vi "Untitled 1.vi"() -> ()   [LabVIEW 2020]
panel:
  in  "Einzel":dbl(slide) scale=0.0..-10000.0
  in  "wisman test":dbl(slide) scale=0.0..10000.0
  in  "stop":bool
  out "einzel":dbl(graph)
  out "Einzel readback":dbl
  out "wisman":dbl(graph)
  out "readback":dbl
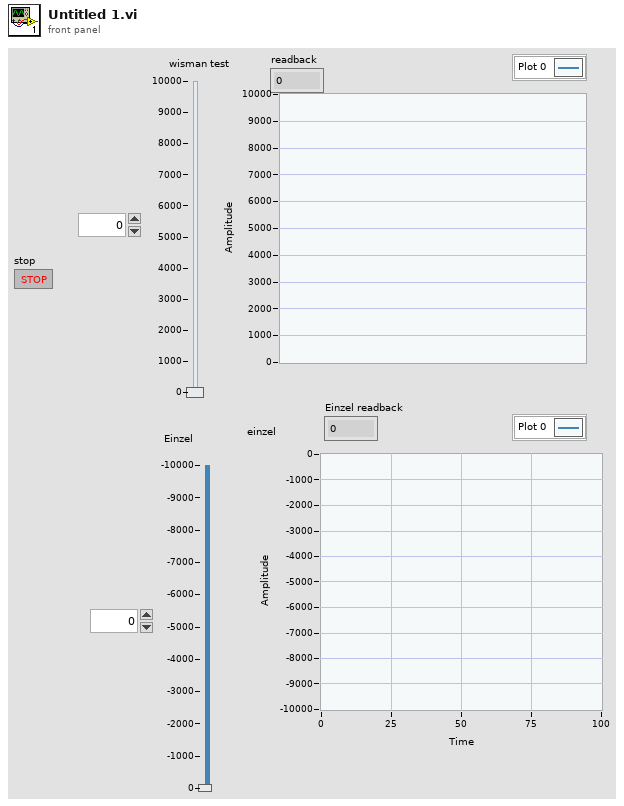
[diagram p1: front panel]
types:
  T1 = enum16{"open", "replace", "create", "open or create", "replace or create", "replace or create with confirmation"}
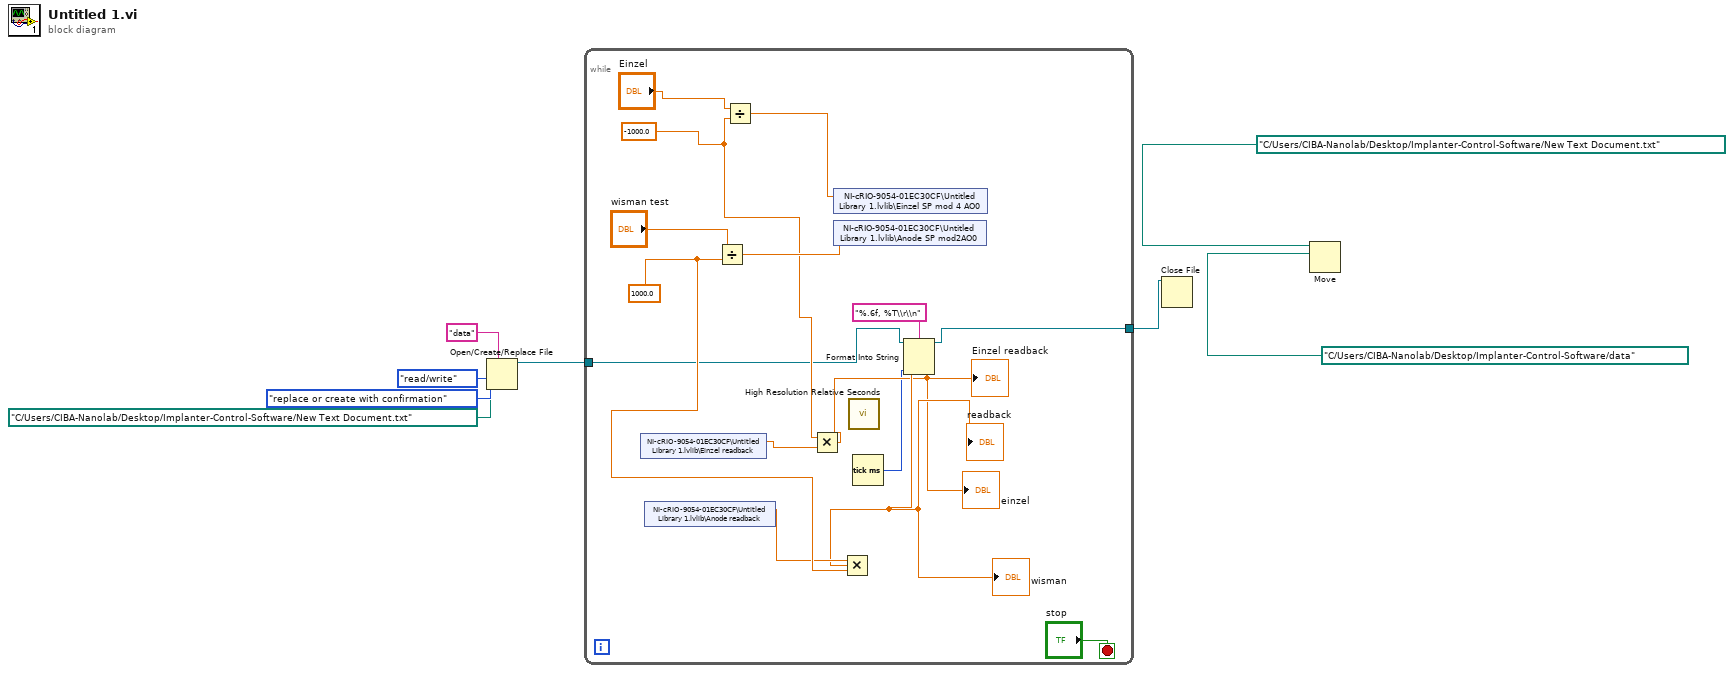
[diagram p0: block diagram]
diagram:
  n1 = Open/Create/Replace File(file path (use dialog)=path "C:/Users/CIBA-Nanolab/Desktop/Implanter-Control-Software/New Text Document.txt", prompt="data", operation (0:open)=T1."replace or create with confirmation", access (0:read/write)=enum16{"read/write", "read-only", "write-only"}."read/write") -> (refnum out=w3:refnum<file>)  [unwired: 2 in, 2 out]
  n2 = while {
    tunnel: [w14] -> w4
    tunnel: w3 -> [w9]
    stop <- "stop" stop-if-true
    w16 = -1000.0
    w18 = 1000.0
    n3 = shared-variable "NI-cRIO-9054-01EC30CF\\Untitled Library 1.lvlib\\Einzel readback"() -> (w15:dbl)  [unwired: 1 in, 1 out]
    n4 = shared-variable "NI-cRIO-9054-01EC30CF\\Untitled Library 1.lvlib\\Anode readback"() -> (w17:dbl)  [unwired: 1 in, 1 out]
    n5 = Divide(x="wisman test", y=w18) -> (x/y=w21:dbl)
    n6 = Divide(x="Einzel", y=w16) -> (x/y=w19:dbl)
    n7 = Multiply(x=w16, y=w15) -> (x*y=→"Einzel readback" →"einzel":dbl)
    n8 = shared-variable "NI-cRIO-9054-01EC30CF\\Untitled Library 1.lvlib\\Einzel SP mod 4 AO0"(w19) -> ()  [unwired: 1 in, 1 out]
    n9 = shared-variable "NI-cRIO-9054-01EC30CF\\Untitled Library 1.lvlib\\Anode SP mod2AO0"(w21) -> ()  [unwired: 1 in, 1 out]
    n10 = Multiply(x=w17, y=w18) -> (x*y=w12:dbl)
    "readback" <- w12
    "wisman" <- w12
    n11 = call <vilib>:"High Resolution Relative Seconds.vi"() -> ()  [unwired: 1 out]
    n12 = Tick Count (ms)() -> (millisecond timer value=w10:u32)
    n13 = Format Into String(format string="%.6f, %T\\r\\n", initial string=w9, w12, w10) -> (resulting string=w14:refnum<file>)  [unwired: 1 in, 1 out]
  }
  n14 = Close File(refnum=w4) -> ()  [unwired: 1 in, 2 out]
  n15 = Move(source path=path "C:/Users/CIBA-Nanolab/Desktop/Implanter-Control-Software/New Text Document.txt", 10:path "C:/Users/CIBA-Nanolab/Desktop/Implanter-Control-Software/data" ("target path (use dialog)")) -> ()  [unwired: 3 in, 3 out]
